vi "Get Output Array.vi"(8 "error in":errorcluster, 11 "Device Ref in":T1 format="%.0x") -> (0 "error out":errorcluster, 3 "Array":string[](array[string]))   [LabVIEW 2021, in "G5 Regatron Custom Device Engine.lvlib"]
uses:
  G5 Regatron Custom Device Engine.lvlib
  <vilib>/NI VeriStand/Custom Device API/Custom Device Item Ref.ctl
  <vilib>/NI VeriStand/Custom Device API/Custom Device API.lvlib
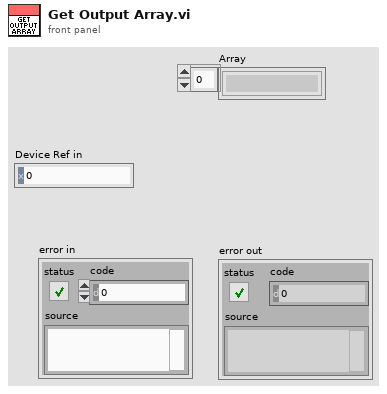
[diagram p1: front panel]
types:
  T1 = typedef "Custom Device API.lvlib/Custom Device Item Ref.ctl" = u64
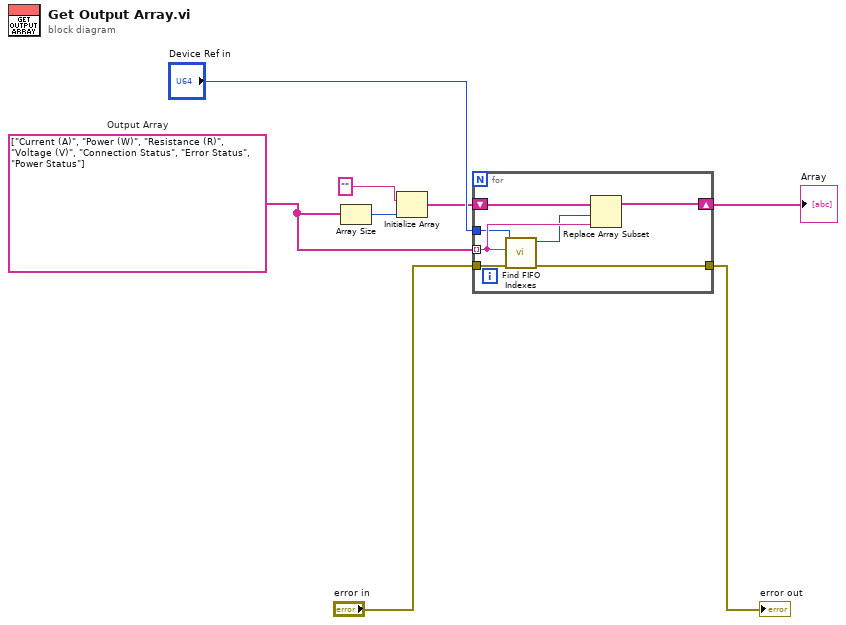
[diagram p0: block diagram]
diagram:
  w5 = string[] ["Current (A)", "Power (W)", "Resistance (R)", "Voltage (V)", "Connection Status", "Error Status", "Power Status"]  # Output Array
  n1 = Array Size(array=w5) -> (size(s)=w2:i32)
  n2 = Initialize Array("" ("String"), w2) -> (w4:string[])
  n3 = for {
    tunnel: w5 -> [w11] mode=indexing
    tunnel: "error in" -> [w15]
    tunnel: [w14] -> w6
    shift-right: [w12] -> w7
    shift-left: w4 -> [w13]
    tunnel: "Device Ref in" -> [w9]
    n4 = call "Find FIFO Indexes.vi"("error in"=w15, "Item Name"=w11, "Custom Device Ref in"=w9) -> ("error out"=w14:errorcluster, "Index"=w10:i32)  [unwired: 7 in]
    n5 = Replace Array Subset(array=w13, new element=w11, index=w10) -> (w12:string[])
  }
  "Array" <- w7
  "error out" <- w6
